vi "Convert Array to CameraOption.vi"(1 "CAMERAOPTIONS Data":u32[](array[numeric])) -> (0 "CAMERAOPTIONS":T1 {"VideoSystem" items=["VIDEOSYS_NTSC"=0, "VIDEOSYS_PAL"=1, "VIDEOSYS_720P60"=4, "VIDEOSYS_720P59DOT9"=12, "VIDEOSYS_720P50"=5, "VIDEOSYS_1080P30"=20, "VIDEOSYS_1080P29DOT9"=28, "VIDEOSYS_1080P25"=21, "VIDEOSYS_1080P24"=36, "VIDEOSYS_1080P23DOT9"=44, "VIDEOSYS_1080I30"=68, "VIDEOSYS_1080I29DOT9"=76, "VIDEOSYS_1080I25"=69, "VIDEOSYS_1080PSF30"=52, "VIDEOSYS_1080PSF29DOT9"=60, "VIDEOSYS_1080PSF25"=53, "VIDEOSYS_1080PSF24"=84, "VIDEOSYS_1080PSF23DOT9"=92]})   [LabVIEW 2013, in "VRI.lvlib"]
uses:
  VRI.lvlib
  _Type Defs/PHCon CAMERAOPTIONS.ctl
  _Type Defs/PhCon VideoSystem.ctl
  _Type Defs/RGBQUAD.ctl
  _Type Defs/PHCon IMRANGE.ctl
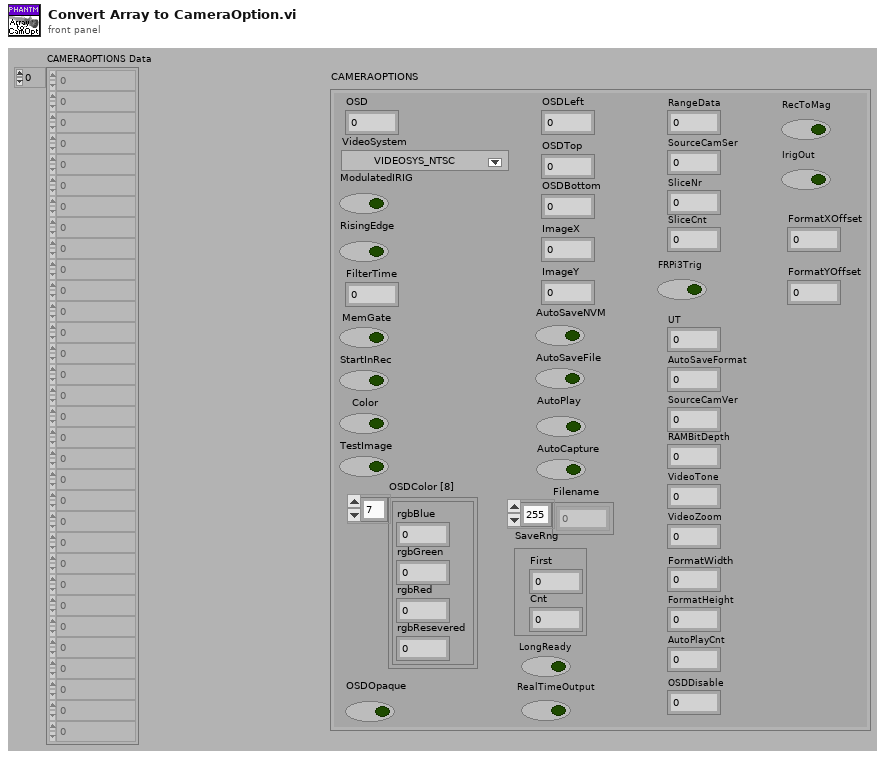
[diagram p1: front panel]
types:
  T1 = typedef "VRI.lvlib/PHCon CAMERAOPTIONS.ctl" = cluster{"OSD":u32, "VideoSystem":T2, "ModulatedIRIG":bool, "RisingEdge":bool, "FilterTime":u32, "MemGate":bool, "StartInRec":bool, "Color":bool, "TestImage":bool, "OSDColor [8]":T3[], "OSDOpaque":bool, "OSDLeft":i32, "OSDTop":i32, "OSDBottom":i32, "ImageX":i32, "ImageY":i32, "AutoSaveNVM":bool, "AutoSaveFile":bool, "AutoPlay":bool, "AutoCapture":bool, "Filename":u8[], "SaveRng":T4, "LongReady":bool, "RealTimeOutput":bool, "RangeData":u32, "SourceCamSer":u32, "SliceNr":u32, "SliceCnt":u32, "FRPi3Trig":bool, "UT":u32, "AutoSaveFormat":i8, "SourceCamVer":u32, "RAMBitDepth":u32, "VideoTone":i32, "VideoZoom":i32, "FormatWidth":i32, "FormatHeight":i32, "AutoPlayCnt":u32, "OSDDisable":u32, "RecToMag":bool, "IrigOut":bool, "FormatXOffset":i32, "FormatYOffset":i32}
  T2 = typedef "VRI.lvlib/PhCon VideoSystem.ctl" = u32
  T3 = typedef "VRI.lvlib/RGBQUAD.ctl" = cluster{"rgbBlue":u8, "rgbGreen":u8, "rgbRed":u8, "rgbResevered":u8}
  T4 = typedef "VRI.lvlib/PHCon IMRANGE.ctl" = cluster{"First":i32, "Cnt":u32}
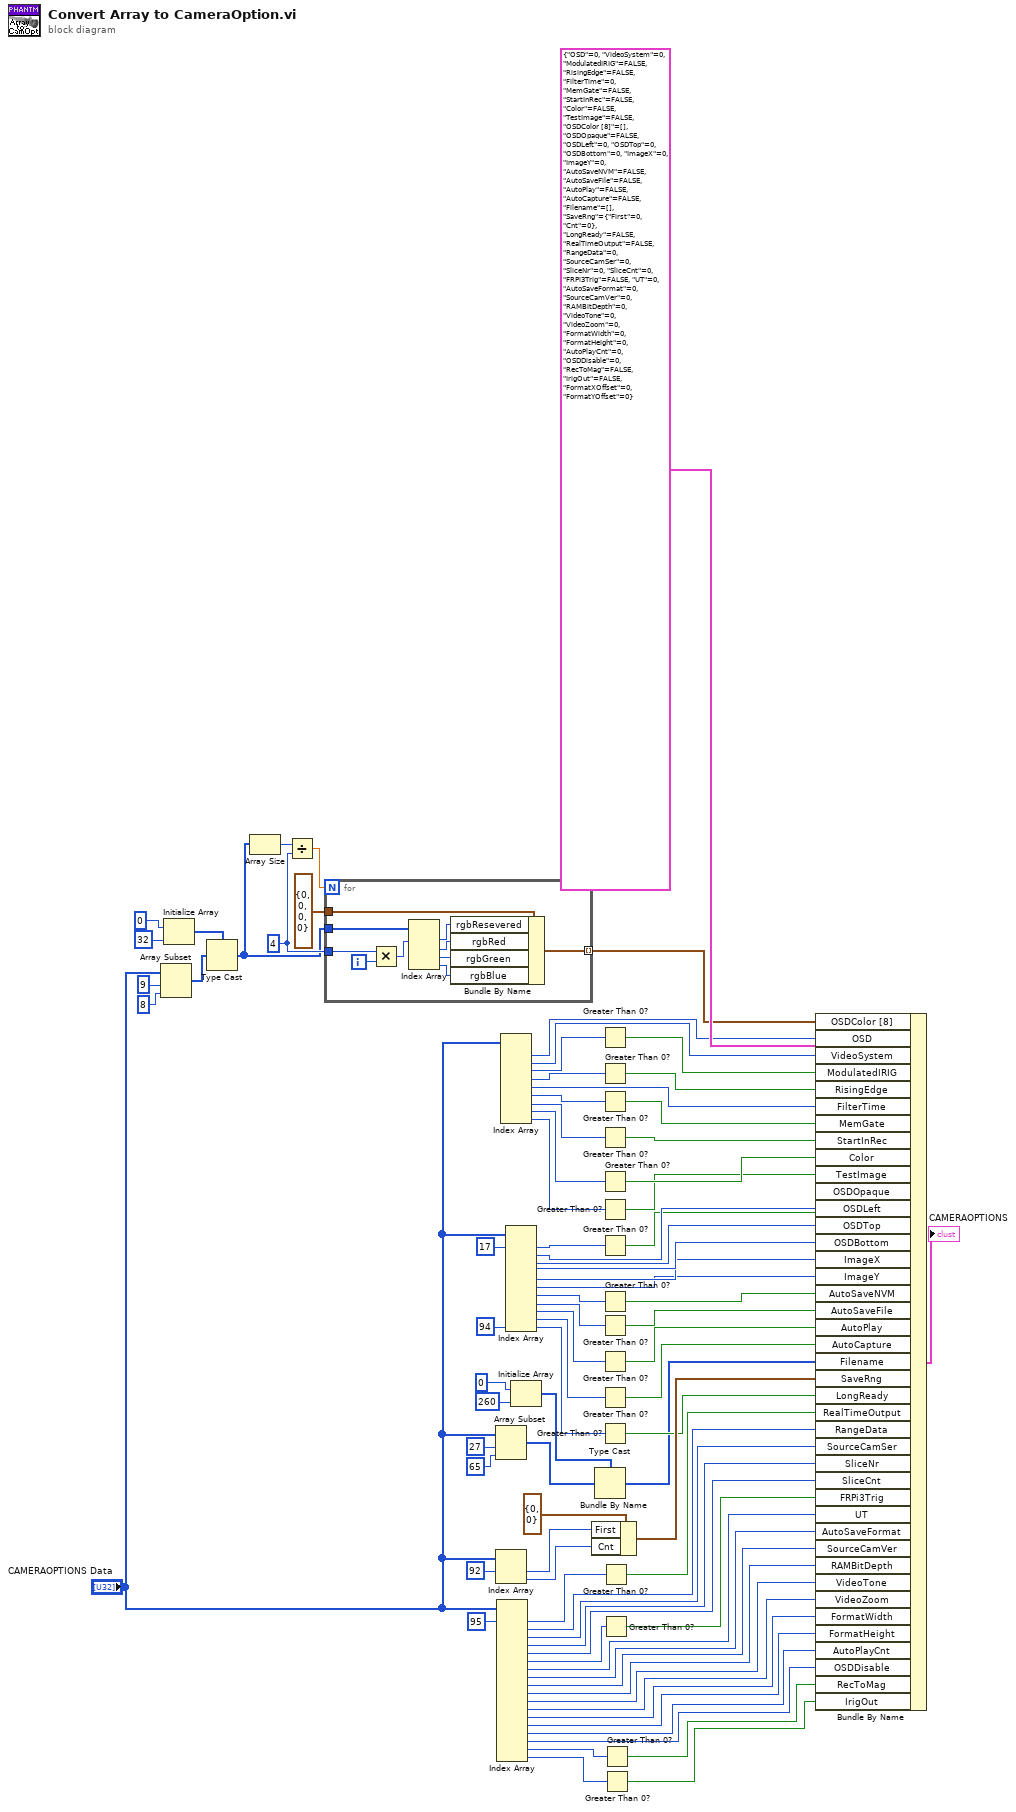
[diagram p0: block diagram]
diagram:
  w41 = 4 ("y")
  n1 = Array Subset(array="CAMERAOPTIONS Data", index=9, length=8) -> (w34:u32[])
  n2 = Initialize Array(u8 0 ("element"), 32 ("dimension size")) -> (w31:u8[])
  n3 = Type Cast(type=w31, x=w34) -> (*(type *) &x=w30:u8[])
  n4 = Array Size(array=w30) -> (size(s)=w44:i32)
  n5 = Divide(x=w44, y=w41) -> (x/y=w45:dbl)
  n6 = for {
    N: w45 -> [_]
    tunnel: w30 -> [w92]
    tunnel: T3 {"rgbBlue"=0, "rgbGreen"=0, "rgbRed"=0, "rgbResevered"=0} ("RGBQUAD") -> [w94]
    tunnel: [w93] -> w42 mode=indexing
    tunnel: w41 -> [w86]
    i -> [w85]
    n7 = Multiply(x=w86, y=w85) -> (x*y=w87:i32)
    n8 = Index Array(array=w92, index #1=w87) -> (element #1=w91:u8, element #2=w90:u8, element #3=w89:u8, element #4=w88:u8)  [unwired: 3 in]
    n9 = Bundle By Name(cluster=w94, "rgbResevered"=w91, "rgbRed"=w90, "rgbGreen"=w89, "rgbBlue"=w88) -> (w93:T3)
  }
  n10 = Array Subset(array="CAMERAOPTIONS Data", index=27, length=65) -> (w26:u32[])
  n11 = Index Array(array="CAMERAOPTIONS Data", index #1=92 ("index")) -> (element #1=w38:u32, element #2=w37:u32)  [unwired: 1 in]
  n12 = Index Array(array="CAMERAOPTIONS Data", index #1=95 ("index")) -> (element #1=w23:u32, element #2=w20:u32, element #3=w19:u32, element #4=w18:u32, element #5=w17:u32, element #6=w16:u32, element #7=w14:u32, element #8=w13:u32, element #9=w12:u32, element #10=w11:u32, element #11=w10:u32, element #12=w9:u32, element #13=w8:u32, element #14=w7:u32, element #15=w6:u32, element #16=w5:u32, element #17=w4:u32, element #18=w3:u32)  [unwired: 17 in]
  n13 = Index Array(array="CAMERAOPTIONS Data") -> (element #1=w35:u32, element #2=w84:u32, element #3=w83:u32, element #4=w82:u32, element #5=w81:u32, element #6=w80:u32, element #7=w79:u32, element #8=w78:u32, element #9=w77:u32)  [unwired: 9 in]
  n14 = Index Array(array="CAMERAOPTIONS Data", index #1=17 ("index"), index #11=94 ("index")) -> (element #1=w73:u32, element #2=w72:u32, element #3=w71:u32, element #4=w70:u32, element #5=w69:u32, element #6=w68:u32, element #7=w67:u32, element #8=w46:u32, element #9=w66:u32, element #10=w65:u32, element #11=w62:u32)  [unwired: 9 in]
  n15 = Initialize Array(u8 0 ("element"), 260 ("dimension size")) -> (w27:u8[])
  n16 = Bundle By Name(cluster=T4 {"First"=0, "Cnt"=0} ("SaveRng"), "First"=w38, "Cnt"=w37) -> (w39:T4)
  n17 = Type Cast(type=w27, x=w26) -> (*(type *) &x=w25:u8[])
  n18 = Greater Than 0?(x=w83) -> (x > 0?=w57:bool)
  n19 = Greater Than 0?(x=w82) -> (x > 0?=w56:bool)
  n20 = Greater Than 0?(x=w80) -> (x > 0?=w55:bool)
  n21 = Greater Than 0?(x=w79) -> (x > 0?=w54:bool)
  n22 = Greater Than 0?(x=w78) -> (x > 0?=w53:bool)
  n23 = Greater Than 0?(x=w77) -> (x > 0?=w52:bool)
  n24 = Greater Than 0?(x=w73) -> (x > 0?=w51:bool)
  n25 = Greater Than 0?(x=w67) -> (x > 0?=w47:bool)
  n26 = Greater Than 0?(x=w46) -> (x > 0?=w48:bool)
  n27 = Greater Than 0?(x=w66) -> (x > 0?=w49:bool)
  n28 = Greater Than 0?(x=w65) -> (x > 0?=w50:bool)
  n29 = Greater Than 0?(x=w62) -> (x > 0?=w36:bool)
  n30 = Greater Than 0?(x=w23) -> (x > 0?=w21:bool)
  n31 = Greater Than 0?(x=w16) -> (x > 0?=w15:bool)
  n32 = Greater Than 0?(x=w4) -> (x > 0?=w2:bool)
  n33 = Greater Than 0?(x=w3) -> (x > 0?=w1:bool)
  n34 = Bundle By Name(cluster=T1 {"OSD"=0, "VideoSystem"=0, "ModulatedIRIG"=FALSE, "RisingEdge"=FALSE, "FilterTime"=0, "MemGate"=FALSE, "StartInRec"=FALSE, "Color"=FALSE, "TestImage"=FALSE, "OSDColor [8]"=[], "OSDOpaque"=FALSE, "OSDLeft"=0, "OSDTop"=0, "OSDBottom"=0, "ImageX"=0, "ImageY"=0, "AutoSaveNVM"=FALSE, "AutoSaveFile"=FALSE, "AutoPlay"=FALSE, "AutoCapture"=FALSE, "Filename"=[], "SaveRng"={"First"=0, "Cnt"=0}, "LongReady"=FALSE, "RealTimeOutput"=FALSE, "RangeData"=0, "SourceCamSer"=0, "SliceNr"=0, "SliceCnt"=0, "FRPi3Trig"=FALSE, "UT"=0, "AutoSaveFormat"=0, "SourceCamVer"=0, "RAMBitDepth"=0, "VideoTone"=0, "VideoZoom"=0, "FormatWidth"=0, "FormatHeight"=0, "AutoPlayCnt"=0, "OSDDisable"=0, "RecToMag"=FALSE, "IrigOut"=FALSE, "FormatXOffset"=0, "FormatYOffset"=0} ("CAMERAOPTIONS"), "OSDColor [8]"=w42, "OSD"=w35, "VideoSystem"=w84, "ModulatedIRIG"=w57, "RisingEdge"=w56, "FilterTime"=w81, "MemGate"=w55, "StartInRec"=w54, "Color"=w53, "TestImage"=w52, "OSDOpaque"=w51, "OSDLeft"=w72, "OSDTop"=w71, "OSDBottom"=w70, "ImageX"=w69, "ImageY"=w68, "AutoSaveNVM"=w47, "AutoSaveFile"=w48, "AutoPlay"=w49, "AutoCapture"=w50, "Filename"=w25, "SaveRng"=w39, "LongReady"=w36, "RealTimeOutput"=w21, "RangeData"=w20, "SourceCamSer"=w19, "SliceNr"=w18, "SliceCnt"=w17, "FRPi3Trig"=w15, "UT"=w14, "AutoSaveFormat"=w13, "SourceCamVer"=w12, "RAMBitDepth"=w11, "VideoTone"=w10, "VideoZoom"=w9, "FormatWidth"=w8, "FormatHeight"=w7, "AutoPlayCnt"=w6, "OSDDisable"=w5, "RecToMag"=w2, "IrigOut"=w1) -> (→"CAMERAOPTIONS":T1)
